vi "MIPI RFFE Read Waveform_no harware compare.vi"(0 "Data":T1 {"Register" format="%.0x"; "Slave Address" max=15 format="%.0x"}, 1 "Ext_Read_Num_Reg":u8, 2 "Readback Speed":enum16{"Full Speed", "Half Speed"}(ring), 5 "Configuratation":T2={"Samples to Allocate"=10000, "Oversample Factor"=1, "Clock Channel"=enum."0", "Data Channel"=enum."1"} {"Oversample Factor" min=1 max=254; "Samples to Allocate" min=1}, 11 "error in (no error)":errorcluster) -> (6 "Waveform Graph":digitalwaveform(graph), 15 "error out":errorcluster)   [LabVIEW 2013]
uses:
  Ctrls/Configuration.ctl
  Ctrls/ClockDataChannels.ctl
  Ctrls/RegReadWrite.ctl
  Ctrls/ExtendedRegReadWrite.ctl
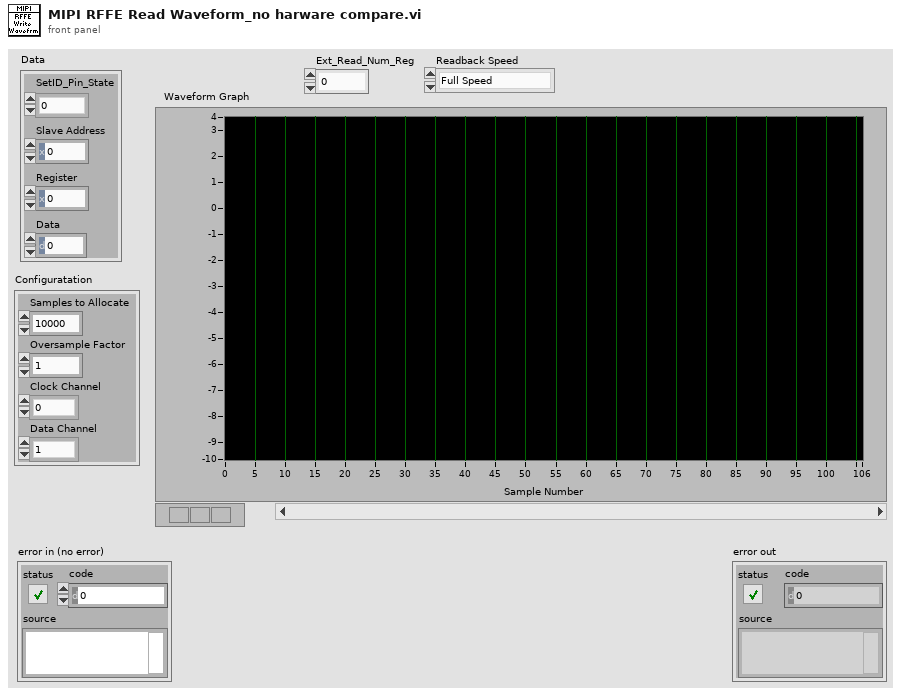
[diagram p1: front panel]
types:
  T1 = typedef "RegReadWrite.ctl" = cluster{"Slave Address":u8, "Register":u8, "Data":u8, "SetID_Pin_State":enum16{"0", "1", "Z"}}
  T2 = typedef "Configuration.ctl" = cluster{"Samples to Allocate":i32, "Oversample Factor":u8, "Clock Channel":T3, "Data Channel":T3}
  T3 = typedef "ClockDataChannels.ctl" = enum16{"0", "1"}
  T4 = typedef "RFFE_Data.ctl" = cluster{"Clock Channel":T3, "Data Channel":T3, "Oversample Factor":u8, "Zero Array":u8[], "One Array":u8[], "Z Array ":u8[], "H Array":u8[], "L Array":u8[], "X Array":u8[], "Toggle (high to low)":u8[]}
  T5 = typedef "ExtendedRegReadWrite.ctl" = cluster{"Slave Address":u8, "Register":u8, "Data":u8[]}
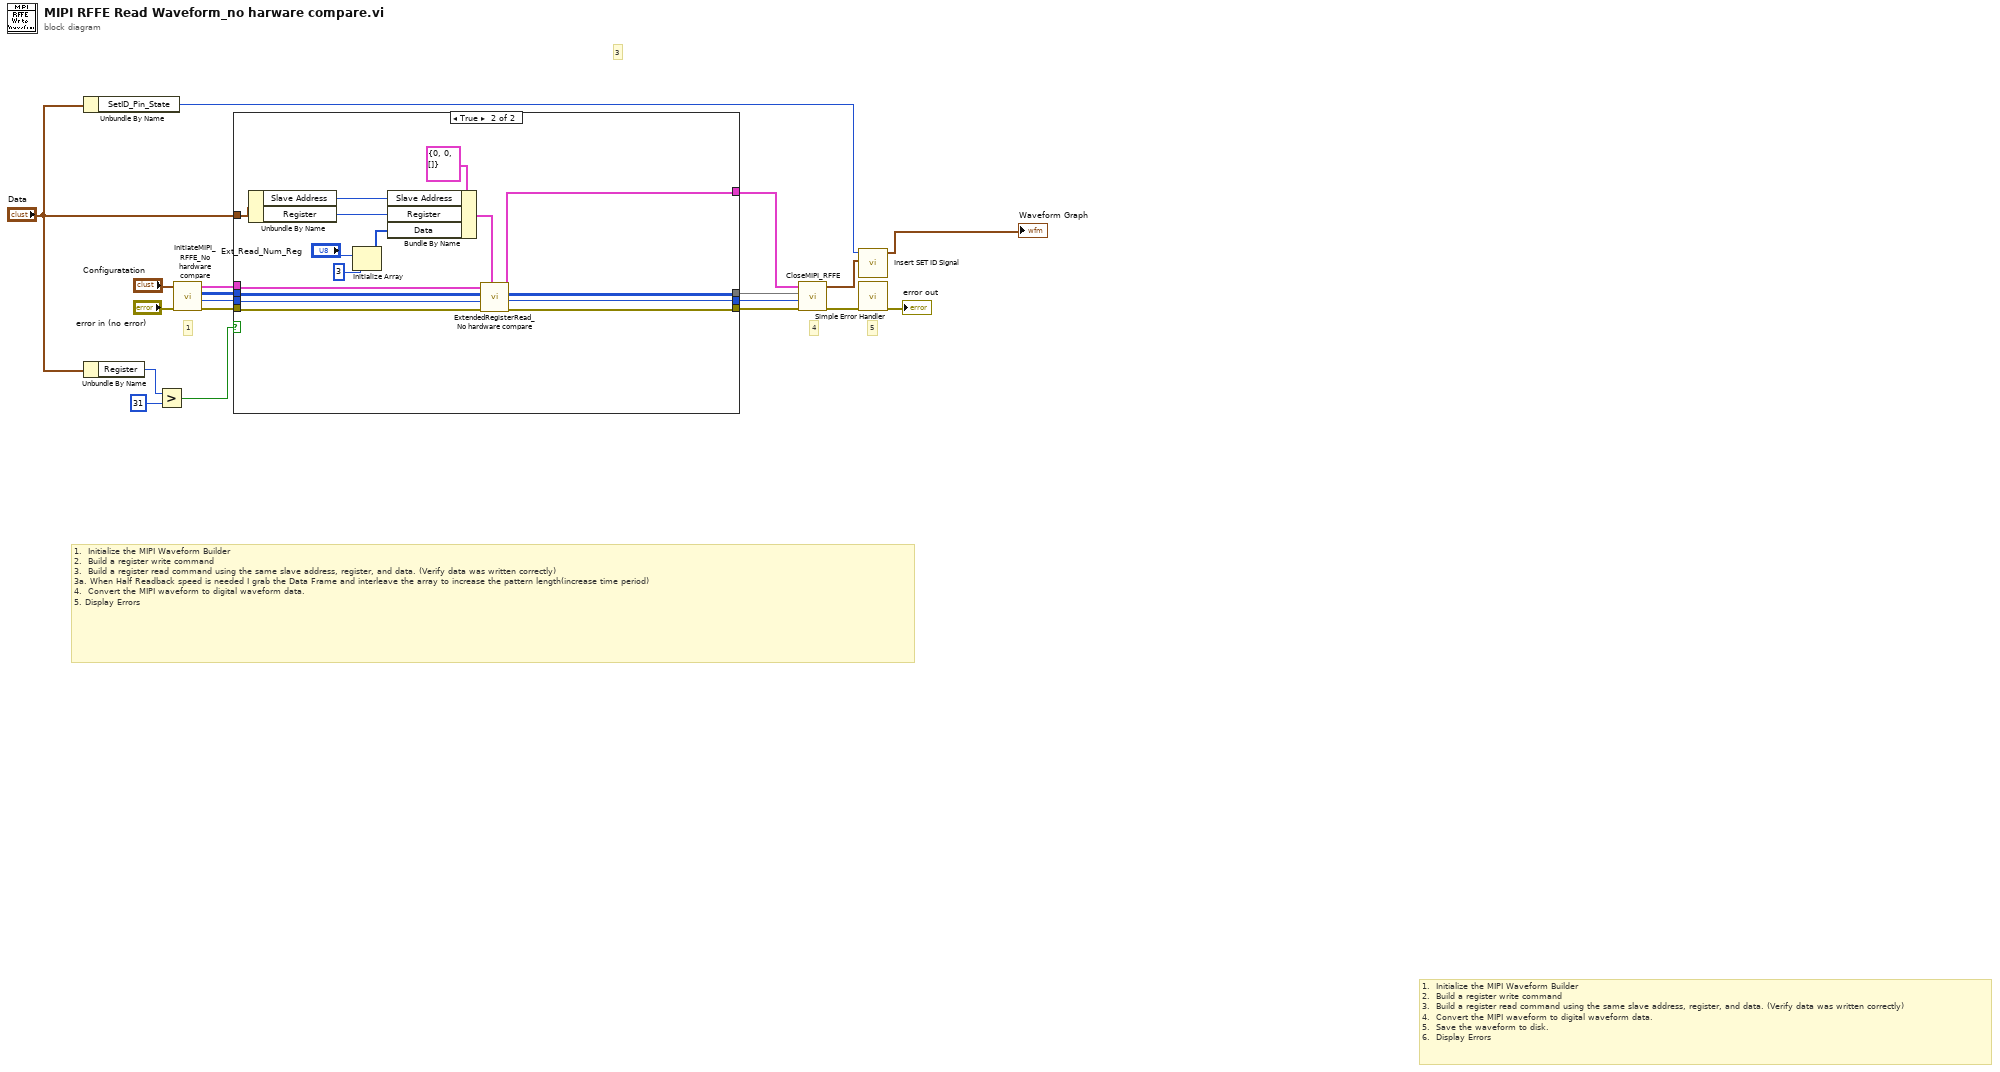
[diagram p0: block diagram]
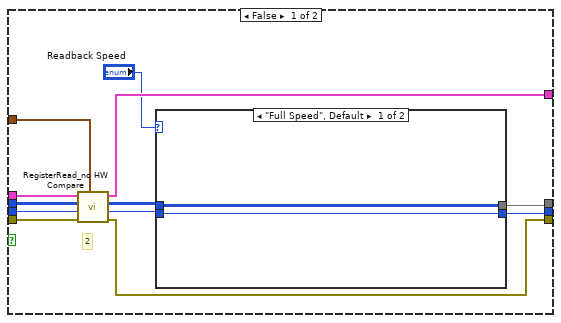
[diagram p2: hidden frame]
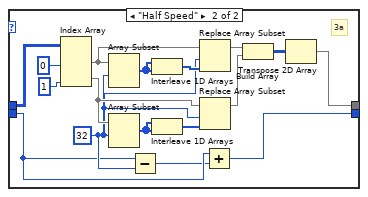
[diagram p3: hidden frame]
diagram:
  # "3"
  # "1.  Initialize the MIPI Waveform Builder\n2.  Build a register write command\n3.  Build a register read command using the same slave address, register, and data. (Verify data was written correctly)\n3a. When Half Readback speed is needed I grab the Data Frame and interleave the array to increase the pattern length(increase time period)\n4.  Convert the MIPI waveform to digital waveform data.\n5. Display Errors"
  # "5"
  # "1.  Initialize the MIPI Waveform Builder\n2.  Build a register write command\n3.  Build a register read command using the same slave address, register, and data. (Verify data was written correctly)\n4.  Convert the MIPI waveform to digital waveform data.\n5.  Save the waveform to disk.\n6.  Display Errors"
  # "4"
  # "1"
  n1 = Unbundle By Name("Data") -> ("SetID_Pin_State"=w1:enum16{"0", "1", "Z"})
  n2 = Unbundle By Name("Data") -> ("Register"=w5:u8)
  n3 = Greater?(x=w5, y=u8 31) -> (0:w3:bool)
  n4 = call "InitiateMIPI_RFFE_No hardware compare.vi"("error in (no error)"="error in (no error)", "Configuratation In"="Configuratation") -> ("error out"=w12:errorcluster, "Number of Samples Out"=w13:i32, "Data Array"=w14:u8[][], "RFFE_Data"=w15:T4)  [unwired: 6 in]
  n5 = case shown="True" w3 {
    tunnel: w15 -> [w31 w65]
    tunnel: w14 -> [w30 w64]
    tunnel: w13 -> [w29 w63]
    tunnel: w12 -> [w28 w66]
    tunnel: [w27 w57] -> w11
    tunnel: [w26 w54] -> w10
    tunnel: [w23 w56] -> w9
    tunnel: [w21 w55] -> w8
    tunnel: "Data" -> [w20 w62]
    frame False {
      # "2"
      n6 = call "RegisterRead_no HW Compare.vi"("Register Read/Write"=w20, "error in (no error)"=w28, "Number of Samples In"=w29, "Data Array"=w30, "RFFE_Data In"=w31) -> ("error out"=w27:errorcluster, "Number of Samples Out out"=w22:i32, "Data Array Out"=w24:u8[][], "RFFE_Data Out"=w26:T4)  [unwired: 2 in, 1 out]
      n7 = case shown="\"Full Speed\", Default" "Readback Speed" {
        tunnel: w24 -> [w33 w39]
        tunnel: [w33 w38] -> w23
        tunnel: w22 -> [w32 w36]
        tunnel: [w32 w34] -> w21
        frame "Full Speed", Default {
        }
        frame "Half Speed" {
          w37 = 32 ("index")
          # "3a"
          n8 = Index Array(array=w39, index (col) #1=0 ("index (row)"), index (col) #2=1 ("index (row)")) -> (element #1=w44:u8[], element #2=w49:u8[])  [unwired: 2 in]
          n9 = Array Subset(array=w44, index=w37) -> (w40:u8[])  [unwired: 1 in]
          n10 = Array Subset(array=w49, index=w37) -> (w41:u8[])  [unwired: 1 in]
          n11 = Subtract(x=w36, y=w37) -> (x-y=w35:i32)
          n12 = Interleave 1D Arrays(w40, w40) -> (w50:u8[])
          n13 = Interleave 1D Arrays(w41, w41) -> (w45:u8[])
          n14 = Replace Array Subset(array=w44, new element=w50, index=w37) -> (w46:u8[])
          n15 = Replace Array Subset(array=w49, new element=w45, index=w37) -> (w48:u8[])
          n16 = Add(x=w36, y=w35) -> (x+y=w34:i32)
          n17 = Build Array(w46, w48) -> (w47:u8[][])
          n18 = Transpose 2D Array(2D array=w47) -> (transposed array=w38:u8[][])
        }
      }
    }
    frame True {
      n19 = Unbundle By Name(w62) -> ("Slave Address"=w60:u8, "Register"=w61:u8)
      n20 = Initialize Array("Ext_Read_Num_Reg", 3 ("dimension size")) -> (w51:u8[])
      n21 = Bundle By Name(cluster=T5 {"Slave Address"=0, "Register"=0, "Data"=[]} ("Extended Read/Write"), "Slave Address"=w60, "Register"=w61, "Data"=w51) -> (w58:T5)
      n22 = call "ExtendedRegisterRead_No hardware compare.vi"("Extended Read/Write"=w58, "error in (no error)"=w66, "Number of Samples In"=w63, "Data Array"=w64, "RFFE_Data In"=w65) -> ("error out"=w57:errorcluster, "Number of Samples Out out"=w55:i32, "Data Array Out"=w56:u8[][], "RFFE_Data Out"=w54:T4)  [unwired: 3 in]
    }
  }
  n23 = call "CloseMIPI_RFFE.vi"("error in (no error)"=w11, "Number of Samples"=w8, "Data Array"=w9, "RFFE_Data"=w10) -> ("error out"=w18:errorcluster, "Digital Waveform"=w7:digitalwaveform)  [unwired: 6 in]
  n24 = call "Insert SET ID Signal.vi"("Digital Waveform Graph"=w7, "SetID_Pin_State"=w1) -> ("Digital Waveform Graph 2"=→"Waveform Graph":digitalwaveform)  [unwired: 9 in]
  n25 = call <vilib>:"Simple Error Handler.vi"("error in (no error)"=w18) -> ("error out"=→"error out":errorcluster)  [unwired: 4 in, 4 out]
